vi "Teardown.vi"(7 "Actor in":refnum<class "Actor.lvclass">, 11 "Msg State in":refnum<class "Msg State.lvclass">) -> (2 "Teardown?":bool, 5 "Actor out":refnum<class "Actor.lvclass">)   [LabVIEW 2021, in "jettl.lvlib" / "Msg State.lvclass"]
uses:
  Msg State.lvclass
  Actor/Actor.lvclass
  Msgs/Destroy/Destroy Msg/Destroy Msg.lvclass
  C:/git/jettl/src/jettl/Msg/Msg.lvclass
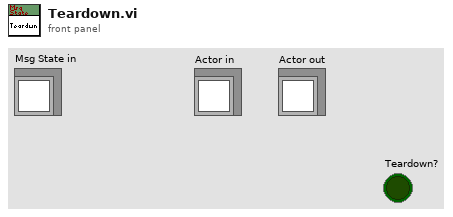
[diagram p1: front panel]
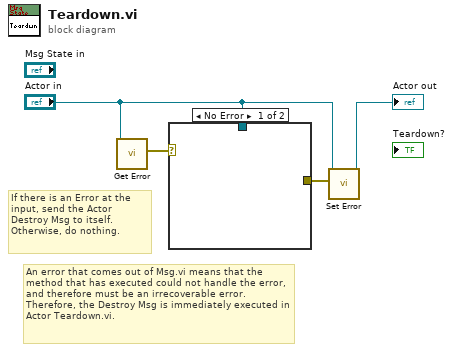
[diagram p0: block diagram]
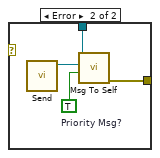
[diagram p2: hidden frame]
diagram:
  # "An error that comes out of Msg.vi means that the method that has executed could not handle the error, and therefore must be an irrecoverable error. Therefore, the Destroy Msg is immediately executed in Actor Teardown.vi."
  # "If there is an Error at the input, send the Actor Destroy Msg to itself. Otherwise, do nothing."
  n1 = call-dynamic "Get Error.vi"("Actor in"="Actor in") -> ("Error"=w4:errorcluster)  [unwired: 10 in]
  n2 = case shown="No Error" w4 {
    tunnel: "Actor in" -> [_ w8]
    tunnel: [_ w5] -> w3
    frame No Error {
    }
    frame Error {
      w6 = TRUE  # Priority Msg?
      n3 = call "Send.vi"() -> ("Destroy Msg out"=w7:refnum<class "Destroy Msg.lvclass">)  [unwired: 11 in]
      n4 = call-dynamic "Msg To Self.vi"("Priority Msg?"=w6, "Msg"=w7, "Actor in"=w8) -> ("error out"=w5:errorcluster)  [unwired: 8 in]
    }
  }
  n5 = call-dynamic "Set Error.vi"("Error"=w3, "Set Error in"="Actor in") -> ("Set Error out"=→"Actor out":refnum<class "Actor.lvclass">)  [unwired: 9 in]
